vi "crearMatrizPosiciones.vi"() -> (1 "posPiezaCuatro":i32[][](array[numeric]), 2 "posPiezaDos":i32[][](array[numeric]), 3 "posPiezaCinco":i32[](array[numeric]), 4 "posPiezaTres":i32[][](array[numeric]), 5 "posPiezaUno":i32[][](array[numeric]))   [LabVIEW 2020]
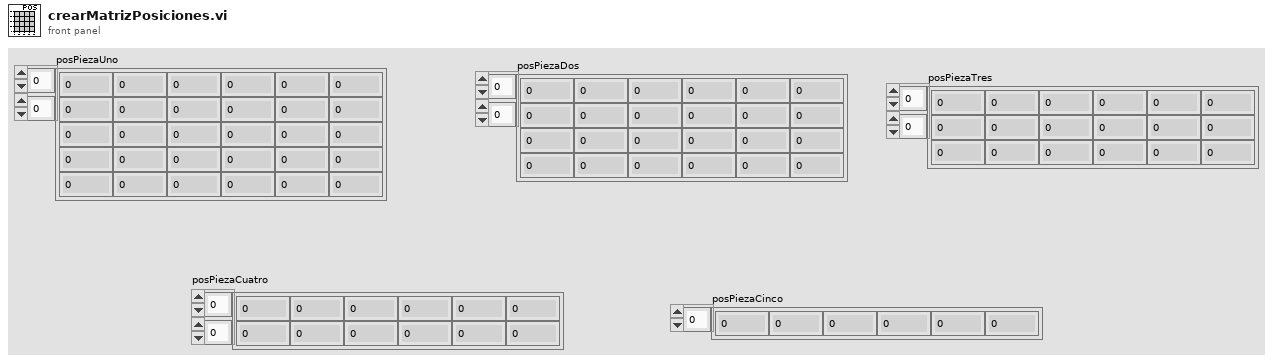
[diagram p1: front panel]
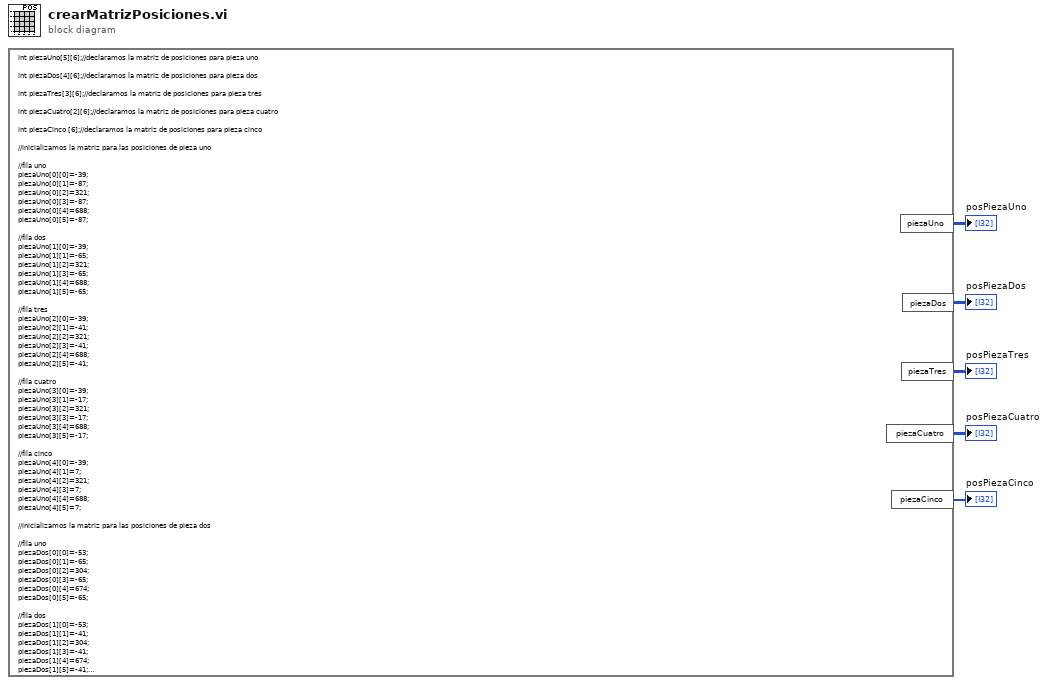
[diagram p0: block diagram]
diagram:
  n1 = formula code="int piezaUno[5][6];//declaramos la matriz de posiciones para pieza uno\n\nint piezaDos[4][6];//declaramos la matriz de posiciones para pieza dos\n\nint piezaTres[3][6];//declaramos la matriz de posiciones para pieza tres\n\nint piezaCuatro[2][6];//declaramos la matriz de posiciones para pieza cuatro\n\nint piezaCinco [6];//declaramos la matriz de posiciones para pieza cinco\n\n//inicializamos la matriz para las posiciones de pieza uno\n\n//fila uno\npiezaUno[0][0]=-39;\npiezaUno[0][1]=-87;\npiezaUno[0][2]=321;\npiezaUno[0][3]=-87;\npiezaUno[0][4]=688;\npiezaUno[0][5]=-87;\n\n//fila dos\npiezaUno[1][0]=-39;\npiezaUno[1][1]=-65;\npiezaUno[1][2]=321;\npiezaUno[1][3]=-65;\npiezaUno[1][4]=688;\npiezaUno[1][5]=-65;\n\n//fila tres\npiezaUno[2][0]=-39;\npiezaUno[2][1]=-41;\npiezaUno[2][2]=321;\npiezaUno[2][3]=-41;\npiezaUno[2][4]=688;\npiezaUno[2][5]=-41;\n\n//fila cuatro\npiezaUno[3][0]=-39;\npiezaUno[3][1]=-17;\npiezaUno[3][2]=321;\npiezaUno[3][3]=-17;\npiezaUno[3][4]=688;\npiezaUno[3][5]=-17;\n\n//fila cinco\npiezaUno[4][0]=-39;\npiezaUno[4][1]=7;\npiezaUno[4][2]=321;\npiezaUno[4][3]=7;\npiezaUno[4][4]=688;\npiezaUno[4][5]=7;\n\n//inicializamos la matriz para las posiciones de pieza dos\n\n//fila uno\npiezaDos[0][0]=-53;\npiezaDos[0][1]=-65;\npiezaDos[0][2]=304;\npiezaDos[0][3]=-65;\npiezaDos[0][4]=674;\npiezaDos[0][5]=-65;\n\n//fila dos\npiezaDos[1][0]=-53;\npiezaDos[1][1]=-41;\npiezaDos[1][2]=304;\npiezaDos[1][3]=-41;\npiezaDos[1][4]=674;\npiezaDos[1][5]=-41;\n\n//fila tres\npiezaDos[2][0]=-53;\npiezaDos[2][1]=-17;\npiezaDos[2][2]=304;\npiezaDos[2][3]=-17;\npiezaDos[2][4]=674;\npiezaDos[2][5]=-17;\n\n//fila cuatro\npiezaDos[3][0]=-53;\npiezaDos[3][1]=7;\npiezaDos[3][2]=304;\npiezaDos[3][3]=7;\npiezaDos[3][4]=674;\npiezaDos[3][5]=7;\n\n//inicializamos la matriz para las posiciones de pieza tres\n\n//fila uno\npiezaTres[0][0]=-66;\npiezaTres[0][1]=-41;\npiezaTres[0][2]=292;\npiezaTres[0][3]=-41;\npiezaTres[0][4]=661;\npiezaTres[0][5]=-41;\n\n//fila dos\npiezaTres[1][0]=-66;\npiezaTres[1][1]=-17;\npiezaTres[1][2]=292;\npiezaTres[1][3]=-17;\npiezaTres[1][4]=661;\npiezaTres[1][5]=-17;\n\n//fila tres\npiezaTres[2][0]=-66;\npiezaTres[2][1]=7;\npiezaTres[2][2]=292;\npiezaTres[2][3]=7;\npiezaTres[2][4]=661;\npiezaTres[2][5]=7;\n\n//inicializamos la matriz para las posiciones de pieza cuatro\n\n//fila uno\npiezaCuatro[0][0]=-90;\npiezaCuatro[0][1]=-17;\npiezaCuatro[0][2]=274;\npiezaCuatro[0][3]=-17;\npiezaCuatro[0][4]=643;\npiezaCuatro[0][5]=-17;\n\n//fila dos\npiezaCuatro[1][0]=-90;\npiezaCuatro[1][1]=7;\npiezaCuatro[1][2]=274;\npiezaCuatro[1][3]=7;\npiezaCuatro[1][4]=643;\npiezaCuatro[1][5]=7;\n\n//inicializamos la matriz para las posiciones de pieza cuatro\n\n//fila uno\npiezaCinco[0]=-108;\npiezaCinco[1]=7;\npiezaCinco[2]=258;\npiezaCinco[3]=7;\npiezaCinco[4]=625;\npiezaCinco[5]=7;"() -> ("piezaUno"=→"posPiezaUno":i32[][], "piezaDos"=→"posPiezaDos":i32[][], "piezaTres"=→"posPiezaTres":i32[][], "piezaCinco"=→"posPiezaCinco":i32[], "piezaCuatro"=→"posPiezaCuatro":i32[][])
